vi "Check Log Calculation.vi"(0 "VISA resource name":refnum<visa-resource-name>, 5 "Channel (0001)":string="0001", 11 "error in (no error)":errorcluster, 14 "Source (\"\")":string) -> (4 "VISA resource name out":refnum<visa-resource-name>, 6 "Result":bool, 8 "Float Position":i32, 15 "error out":errorcluster)   [LabVIEW 2020, in "Yokogawa GX Series.lvlib"]
doc: "This VI sets the alarm hysteresis for <B>DX1000/DX2000 series</B>.\nThis VI can be used on Basic Setting Mode at the <B>Set Execution Mode.VI</B>.\n\nAlarm settings on computation channels can be specified on models with the /M1 or /PM1 math option.\nAlarm settings on external input channels can be specified on models with the /MC1 external input channel option."
uses:
  <instrlib>/Yokogawa GX Series/Yokogawa GX Series.lvlib
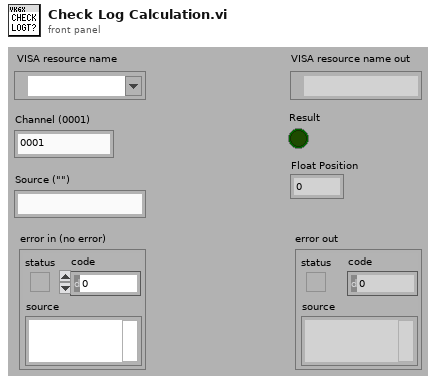
[diagram p1: front panel]
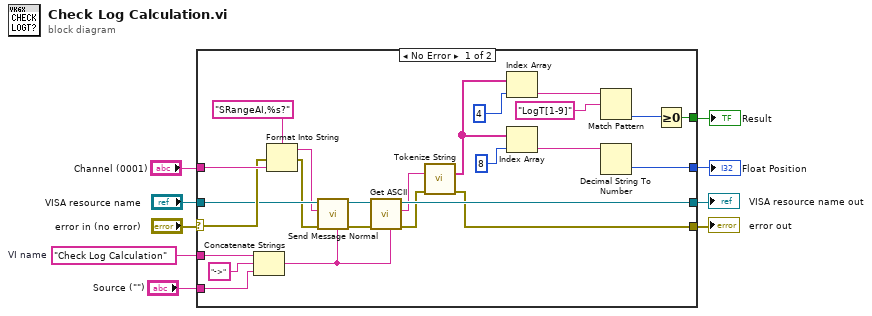
[diagram p0: block diagram]
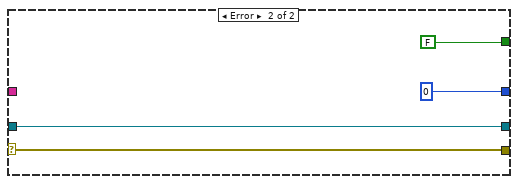
[diagram p2: hidden frame]
diagram:
  w6 = "Check Log Calculation"  # VI name
  n1 = case shown="No Error" "error in (no error)" {
    selector: "error in (no error)" -> [w32 w37]
    tunnel: "VISA resource name" -> [w26 w38]
    tunnel: "Channel (0001)" -> [w33 _]
    tunnel: w6 -> [w31 _]
    tunnel: [w20 w37] -> w5
    tunnel: [w22 w38] -> w4
    tunnel: [w12 FALSE] -> w3
    tunnel: "Source (\"\")" -> [w29 _]
    tunnel: [w10 0] -> w1
    frame No Error {
      n2 = Concatenate Strings(w31, "->", w29) -> (w23:string)
      n3 = Format Into String(format string="SRangeAI,%s?", error in=w32, w33) -> (resulting string=w24:string, error out=w25:errorcluster)  [unwired: 1 in]
      n4 = call <instrlib>:"Send Message Normal.vi"("Source (\"\")"=w23, "error in (no error)"=w25, "Send Message (\"\")"=w24, "VISA resource name"=w26) -> ("error out"=w28:errorcluster, "VISA resource name out"=w27:refnum<visa-resource-name>)  [unwired: 5 in, 1 out]
      n5 = call <instrlib>:"Get ASCII.vi"("Source (\"\")"=w23, "error in (no error)"=w28, "VISA resource name"=w27) -> ("error out"=w21:errorcluster, "ASCII Data"=w19:string, "VISA resource name out"=w22:refnum<visa-resource-name>)  [unwired: 6 in]
      n6 = call <instrlib>:"Tokenize String.vi"("String (\"\")"=w19, "Error In"=w21) -> ("Result"=w16:string[], "Error Out"=w20:errorcluster)  [unwired: 12 in]
      n7 = Index Array(array=w16, index=4) -> (element=w15:string)
      n8 = Index Array(array=w16, index=8) -> (element=w11:string)
      n9 = Match Pattern(string=w15, regular expression="LogT[1-9]") -> (offset past match=w13:i32)  [unwired: 1 in, 3 out]
      n10 = Decimal String To Number(string=w11) -> (number=w10:i32)  [unwired: 2 in, 1 out]
      n11 = Greater Or Equal To 0?(x=w13) -> (x >= 0?=w12:bool)
    }
    frame Error {
    }
  }
  "error out" <- w5
  "VISA resource name out" <- w4
  "Result" <- w3
  "Float Position" <- w1
